vi "Write Display Game Board Msg.vi"(10 "Screen Interface.lvlib:Display Game Board Msg.lvclass":refnum<class "Display Game Board Msg.lvclass">, 11 "Screen Interface in":refnum<class "Screen Interface.lvclass">) -> (3 "Screen Interface out":refnum<class "Screen Interface.lvclass">)   [LabVIEW 2017, in "Screen Interface.lvlib" / "Screen Interface.lvclass"]
uses:
  Screen Interface.lvclass
  Screen Interface Messages/Display Game Board Msg/Display Game Board Msg.lvclass
  Screen Interface.lvclass/Screen Interface.ctl
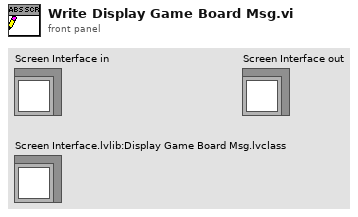
[diagram p1: front panel]
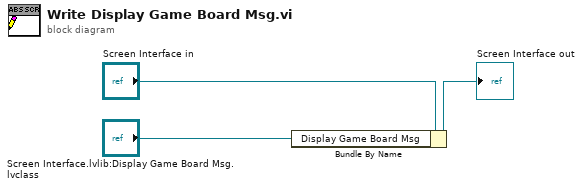
[diagram p0: block diagram]
diagram:
  n1 = Bundle By Name(cluster="Screen Interface in", "Display Game Board Msg"="Screen Interface.lvlib:Display Game Board Msg.lvclass") -> (→"Screen Interface out":refnum<class "Screen Interface.lvclass">)
